vi "L20.vi"() -> ()   [LabVIEW 2012]
panel:
  out "sum":i32
  out "String":string
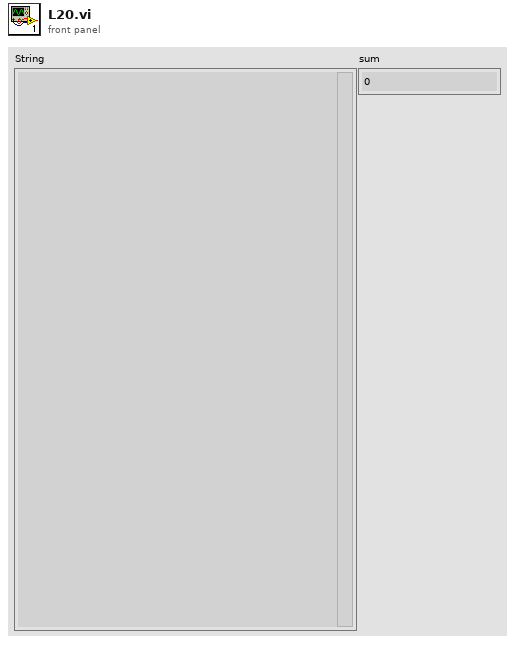
[diagram p1: front panel]
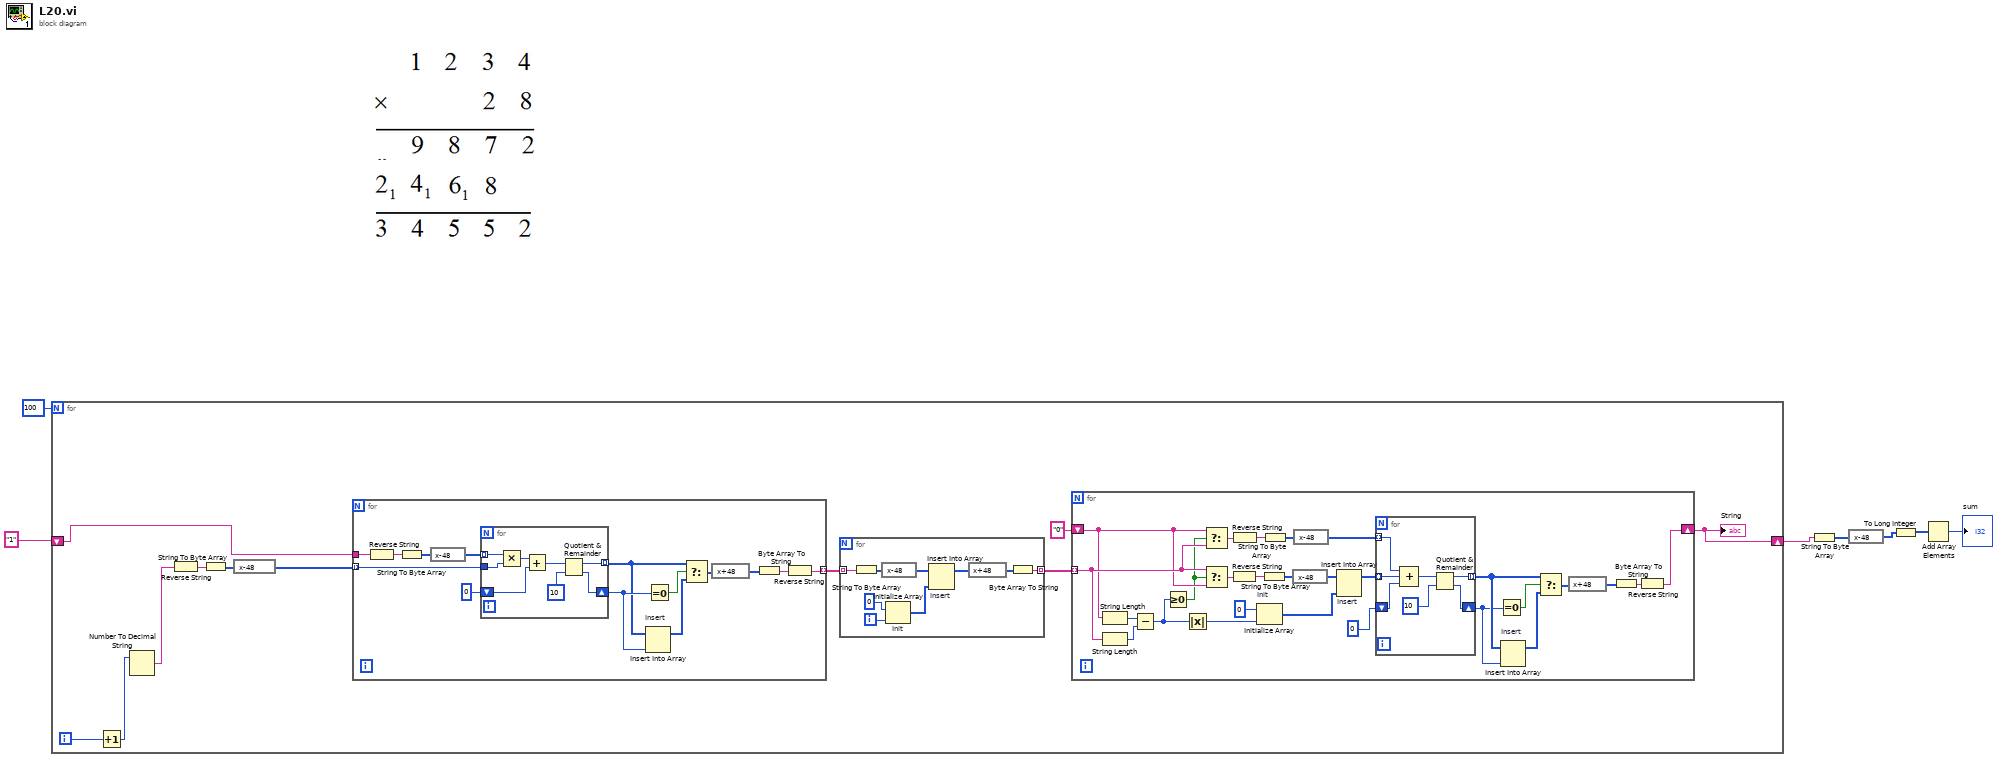
[diagram p0: block diagram]
diagram:
  n1 = for {
    N: 100 -> [_]
    shift-right: [w8] -> w5
    shift-left: "1" -> [w12]
    i -> [w11]
    n2 = Increment(x=w11) -> (x+1=w9:i32)
    n3 = Number To Decimal String(number=w9) -> (decimal integer string=w10:string)  [unwired: 1 in]
    n4 = Reverse String(1:w10) -> (0:w17:string)
    n5 = String To Byte Array(string=w17) -> (unsigned byte array=w18:u8[])
    n6 = expression code="x-48"(w18) -> (w16:u8[])
    n7 = for {
      tunnel: w16 -> [w64] mode=indexing
      tunnel: [w63] -> w14 mode=indexing
      tunnel: w12 -> [w62]
      n8 = Reverse String(1:w62) -> (0:w75:string)
      n9 = String To Byte Array(string=w75) -> (unsigned byte array=w74:u8[])
      n10 = expression code="x-48"(w74) -> (w73:u8[])
      n11 = for {
        tunnel: w73 -> [w83] mode=indexing
        tunnel: [w81] -> w66 mode=indexing
        shift-right: [w80] -> w69
        shift-left: u8 0 -> [w77]
        tunnel: w64 -> [w76]
        n12 = Multiply(x=w83, y=w76) -> (x*y=w79:u8)
        n13 = Add(x=w79, y=w77) -> (x+y=w78:u8)
        n14 = Quotient & Remainder(x=w78, y=u8 10) -> (x-y*floor(x/y)=w81:u8, floor(x/y)=w80:u8)
      }
      n15 = Insert Into Array "Insert"(array=w66, new element=w69) -> (w67:u8[])  [unwired: 1 in]
      n16 = Equal To 0?(x=w69) -> (x = 0?=w68:bool)
      n17 = Select(t=w66, s=w68, f=w67) -> (s? t:f=w65:u8[])
      n18 = expression code="x+48"(w65) -> (w71:u8[])
      n19 = Byte Array To String(unsigned byte array=w71) -> (string=w70:string)
      n20 = Reverse String(1:w70) -> (0:w63:string)
    }
    n21 = for {
      tunnel: w14 -> [w20] mode=indexing
      tunnel: [w19] -> w13 mode=indexing
      i -> [w26]
      n22 = String To Byte Array(string=w20) -> (unsigned byte array=w27:u8[])
      n23 = expression code="x-48"(w27) -> (w24:u8[])
      n24 = Initialize Array "Init"(0 ("element"), w26) -> (w22:i32[])
      n25 = Insert Into Array "Insert"(array=w24, new element=w22) -> (w23:u8[])  [unwired: 1 in]
      n26 = expression code="x+48"(w23) -> (w21:u8[])
      n27 = Byte Array To String(unsigned byte array=w21) -> (string=w19:string)
    }
    n28 = for {
      tunnel: w13 -> [w34] mode=indexing
      shift-right: [w35] -> w8
      shift-left: "0" -> [w33]
      n29 = String Length(string=w33) -> (length=w49:i32)
      n30 = String Length(string=w34) -> (length=w48:i32)
      n31 = Subtract(x=w49, y=w48) -> (x-y=w29:i32)
      n32 = Greater Or Equal To 0?(x=w29) -> (x >= 0?=w32:bool)
      n33 = Absolute Value(x=w29) -> (abs(x)=w28:i32)
      n34 = Select(t=w33, s=w32, f=w34) -> (s? t:f=w31:string)
      n35 = Select(t=w34, s=w32, f=w33) -> (s? t:f=w30:string)
      n36 = Reverse String(1:w30) -> (0:w37:string)
      n37 = Reverse String(1:w31) -> (0:w36:string)
      n38 = Initialize Array "Init"(0 ("element"), w28) -> (w41:i32[])
      n39 = String To Byte Array(string=w37) -> (unsigned byte array=w39:u8[])
      n40 = String To Byte Array(string=w36) -> (unsigned byte array=w38:u8[])
      n41 = expression code="x-48"(w39) -> (w46:u8[])
      n42 = expression code="x-48"(w38) -> (w47:u8[])
      n43 = Insert Into Array "Insert"(array=w46, new element=w41) -> (w42:u8[])  [unwired: 1 in]
      n44 = for {
        tunnel: w42 -> [w57] mode=indexing
        tunnel: [w61] -> w53 mode=indexing
        shift-right: [w59] -> w52
        shift-left: u8 0 -> [w56]
        tunnel: w47 -> [w58] mode=indexing
        n45 = Compound Arithmetic op=ADD(w58, w57, w56) -> (w55:u8)
        n46 = Quotient & Remainder(x=w55, y=u8 10) -> (x-y*floor(x/y)=w61:u8, floor(x/y)=w59:u8)
      }
      n47 = Equal To 0?(x=w52) -> (x = 0?=w51:bool)
      n48 = Insert Into Array "Insert"(array=w53, new element=w52) -> (w50:u8[])  [unwired: 1 in]
      n49 = Select(t=w53, s=w51, f=w50) -> (s? t:f=w54:u8[])
      n50 = expression code="x+48"(w54) -> (w44:u8[])
      n51 = Byte Array To String(unsigned byte array=w44) -> (string=w45:string)
      n52 = Reverse String(1:w45) -> (0:w35:string)
    }
    "String" <- w8
  }
  n53 = String To Byte Array(string=w5) -> (unsigned byte array=w4:u8[])
  n54 = expression code="x-48"(w4) -> (w3:u8[])
  n55 = To Long Integer(number=w3) -> (32bit integer=w2:i32[])
  n56 = Add Array Elements(numeric array=w2) -> (sum=→"sum":i32)
